vi "Autonomous Independent.vi"   [LabVIEW 2013]
doc: "This VI is called when autonomous begins, and will automatically be terminated when autonomous ends. You can carry out timed or sensor driven robot movement independently without needing to return to the caller."
uses:
  Robot Global Data.vi
  <vilib>/Rock Robotics/WPI/RobotDrive/WPI_RobotDriveGetSetRefNum.vi
  <vilib>/Rock Robotics/WPI/RobotDrive/WPI_RobotDriveMecanumDrive_Cartesian.vi
panel:
  # "Be sure to right-click and choose Data Operations>>Make Current Value default if you want to save the array values with the VI"
types:
  T1 = typedef "WPI_RobotDriveDevRef.ctl" = cluster{"DevStatus":errorcluster, "Motors[]":T2[], "Square Inputs":bool, "Max Output":dbl, "Isochronous":bool}
  T2 = typedef "WPI_MotorControlDeviceRef.ctl" = cluster{"DeviceStatus":errorcluster, "Type":enum16{"PWM", "CAN"}, "PWM":cluster{"Digital Module":T3, "PWM Channel":T4, "DeadBand":T5}, "CAN":cluster{"Device Number":u8, "Control Mode":T6, "Semaphore":T7, "Max Vout":dbl}, "Invert":bool, "TransformRef":T8, "InvTransformRef":T8}
  T3 = typedef "FPGA_TypedefDigitalModule.ctl" = enum16{"Digital Module 1", "Digital Module 2"}
  T4 = typedef "FPGA_DIOPWMChannel.ctl" = enum8{"PWM 1", "PWM 2", "PWM 3", "PWM 4", "PWM 5", "PWM 6", "PWM 7", "PWM 8", "PWM 9", "PWM 10", "Invalid"}
  T5 = typedef "WPI_PWMDeadband.ctl" = cluster{"Name":string, "maxPositivePwm":i32, "minPositivePwm":i32, "centerPwm":i32, "maxNegativePwm":i32, "minNegativePwm":i32, "angularRange":u16}
  T6 = typedef "WPI_CANJaguar_ControlMode.ctl" = enum8{"Percent VBus", "Current", "Speed", "Position", "Voltage"}
  T7 = typedef "Semaphore RefNum" = refnum<k1>
  T8 = typedef "WPI_PWMTransform_ConPane.ctl" = refnum<vi>
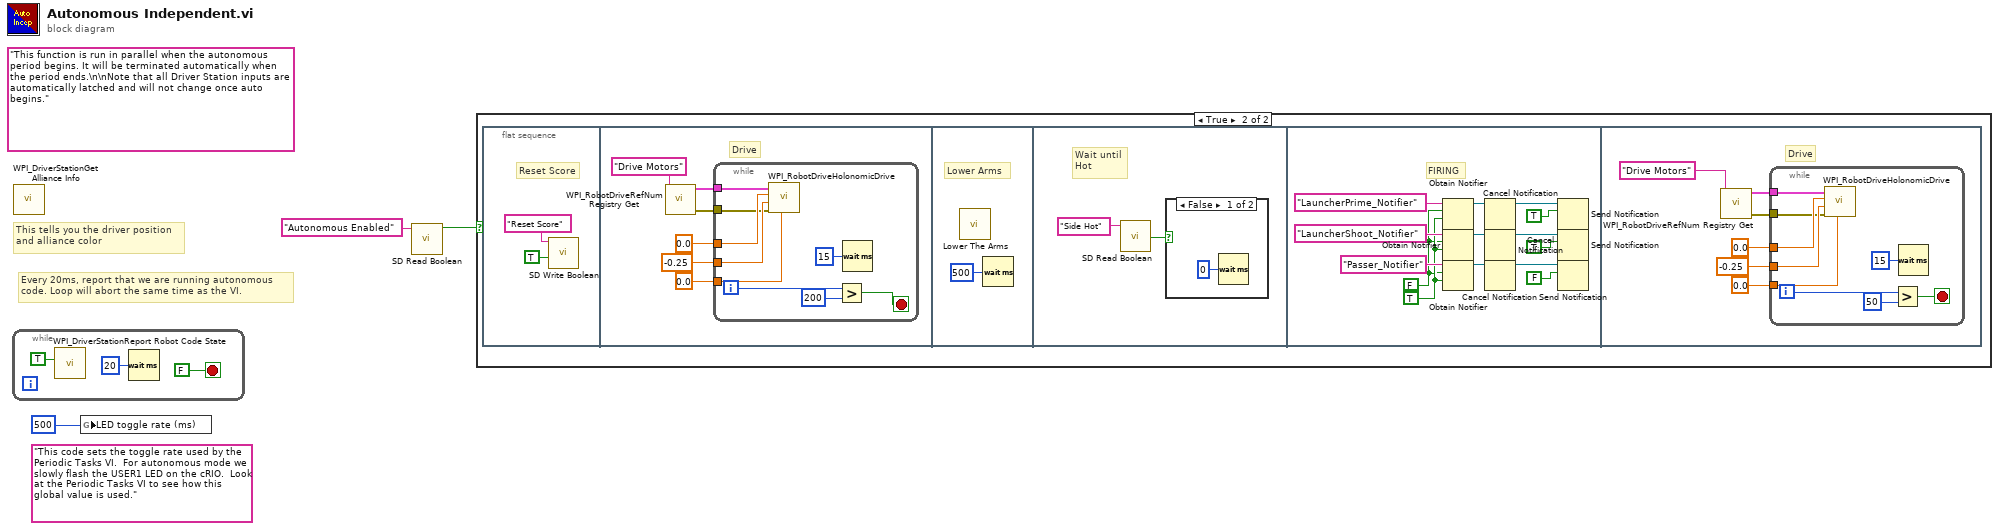
[diagram p0: block diagram]
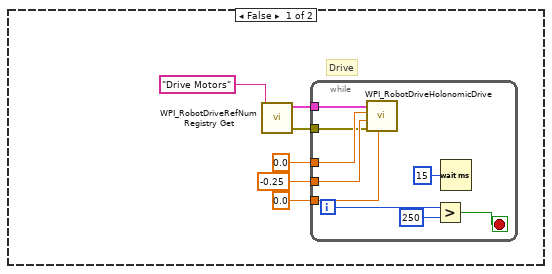
[diagram p2: hidden frame]
diagram:
  (unwired) "This code sets the toggle rate used by the Periodic Tasks VI.  For autonomous mode we slowly flash the USER1 LED on the cRIO.  Look at the Periodic Tasks VI to see how this global value is used."
  (unwired) "This function is run in parallel when the autonomous period begins. It will be terminated automatically when the period ends.\n\nNote that all Driver Station inputs are automatically latched and will not change once auto begins."
  # "Every 20ms, report that we are running autonomous\ncode. Loop will abort the same time as the VI."
  # "This tells you the driver position\nand alliance color"
  n1 = while {
    stop <- FALSE stop-if-true
    n2 = call <vilib>:"WPI_DriverStationReport Robot Code State.vi"("Autonomous"=TRUE) -> ()  [unwired: 10 in, 1 out]
    n3 = Wait (ms)(milliseconds to wait=u32 20) -> ()  [unwired: 1 out]
  }
  n4 = call <vilib>:"WPI_DriverStationGet Alliance Info.vi"() -> ()  [unwired: 12 out]
  n5 = global write "Robot Global Data.vi" "LED toggle rate (ms)"(u32 500 ("LED ms toggle rate")) -> ()
  n6 = call <vilib>:"SD Read Boolean.vi"("Name"="Autonomous Enabled") -> ("Boolean"=w2:bool)  [unwired: 8 in, 2 out]
  n7 = case shown="True" w2 {
    frame False {
      # "Drive"
      n8 = call <vilib>:"WPI_RobotDriveRefNum Registry Get.vi"("refnum name"="Drive Motors") -> ("error out"=w9:errorcluster, "RobotDriveDevRef"=w10:T1)  [unwired: 9 in]
      n9 = while {
        tunnel: -0.25 ("Y") -> [w21]
        tunnel: 0.0 ("X") -> [w20]
        tunnel: w10 -> [w19]
        tunnel: w9 -> [w18]
        tunnel: 0.0 ("Rotation") -> [w17]
        i -> [w15]
        stop <- w13 stop-if-true
        n10 = call-poly <vilib>:"WPI_RobotDriveHolonomicDrive.vi"("Rotation"=w17, "error in (no error)"=w18, "Y"=w21, "X"=w20, "RobotDriveDevRef"=w19) -> ()  [unwired: 4 in, 3 out]
        n11 = Greater?(x=w15, y=250) -> (0:w13:bool)
        n12 = Wait (ms)(milliseconds to wait=u32 15) -> ()  [unwired: 1 out]
      }
    }
    frame True {
      n13 = flat-sequence {
        frame #0 {
          # "Reset Score"
          n14 = call <vilib>:"SD Write Boolean.vi"("Boolean"=TRUE, "Name"="Reset Score") -> ()  [unwired: 8 in, 2 out]
        }
        frame #1 {
          # "Drive"
          n15 = call <vilib>:"WPI_RobotDriveRefNum Registry Get.vi"("refnum name"="Drive Motors") -> ("error out"=w27:errorcluster, "RobotDriveDevRef"=w26:T1)  [unwired: 9 in]
          n16 = while {
            tunnel: -0.25 ("Y") -> [w38]
            tunnel: 0.0 ("X") -> [w37]
            tunnel: w26 -> [w36]
            tunnel: w27 -> [w35]
            tunnel: 0.0 ("Rotation") -> [w34]
            i -> [w32]
            stop <- w30 stop-if-true
            n17 = call-poly <vilib>:"WPI_RobotDriveHolonomicDrive.vi"("Rotation"=w34, "error in (no error)"=w35, "Y"=w38, "X"=w37, "RobotDriveDevRef"=w36) -> ()  [unwired: 4 in, 3 out]
            n18 = Greater?(x=w32, y=200) -> (0:w30:bool)
            n19 = Wait (ms)(milliseconds to wait=u32 15) -> ()  [unwired: 1 out]
          }
        }
        frame #2 {
          # "Lower Arms"
          n20 = call "Lower The Arms.vi"() -> ()  [unwired: 12 in]
          n21 = Wait (ms)(milliseconds to wait=u32 500) -> ()  [unwired: 1 out]
        }
        frame #3 {
          # "Wait until\nHot"
          n22 = call <vilib>:"SD Read Boolean.vi"("Name"="Side Hot") -> ("Boolean"=w40:bool)  [unwired: 8 in, 2 out]
          n23 = case shown="False" w40 {
            frame False {
              n24 = Wait (ms)(milliseconds to wait=u32 0) -> ()  [unwired: 1 out]
            }
            frame True {
            }
          }
        }
        frame #4 {
          w51 = TRUE
          w50 = FALSE
          # "FIRING"
          n25 = Obtain Notifier(name (unnamed)="LauncherPrime_Notifier", notification data type=w50, create if not found? (T)=w51) -> (notifier out=w46:refnum<notifier>)  [unwired: 1 in, 2 out]
          n26 = Obtain Notifier(name (unnamed)="LauncherShoot_Notifier", notification data type=w50, create if not found? (T)=w51) -> (notifier out=w47:refnum<notifier>)  [unwired: 1 in, 2 out]
          n27 = Obtain Notifier(name (unnamed)="Passer_Notifier", notification data type=w50, create if not found? (T)=w51) -> (notifier out=w48:refnum<notifier>)  [unwired: 1 in, 2 out]
          n28 = Cancel Notification(0:w46) -> (8:w45:refnum<notifier>)  [unwired: 1 in, 2 out]
          n29 = Cancel Notification(0:w47) -> (8:w44:refnum<notifier>)  [unwired: 1 in, 2 out]
          n30 = Cancel Notification(0:w48) -> (8:w43:refnum<notifier>)  [unwired: 1 in, 2 out]
          n31 = Send Notification(notification=TRUE, notifier=w45) -> ()  [unwired: 1 in, 2 out]
          n32 = Send Notification(notification=TRUE, notifier=w44) -> ()  [unwired: 1 in, 2 out]
          n33 = Send Notification(notification=FALSE, notifier=w43) -> ()  [unwired: 1 in, 2 out]
        }
        frame #5 {
          # "Drive"
          n34 = call <vilib>:"WPI_RobotDriveRefNum Registry Get.vi"("refnum name"="Drive Motors") -> ("error out"=w59:errorcluster, "RobotDriveDevRef"=w60:T1)  [unwired: 9 in]
          n35 = while {
            tunnel: -0.25 ("Y") -> [w71]
            tunnel: 0.0 ("X") -> [w70]
            tunnel: w60 -> [w69]
            tunnel: w59 -> [w68]
            tunnel: 0.0 ("Rotation") -> [w67]
            i -> [w65]
            stop <- w63 stop-if-true
            n36 = call-poly <vilib>:"WPI_RobotDriveHolonomicDrive.vi"("Rotation"=w67, "error in (no error)"=w68, "Y"=w71, "X"=w70, "RobotDriveDevRef"=w69) -> ()  [unwired: 4 in, 3 out]
            n37 = Greater?(x=w65, y=50) -> (0:w63:bool)
            n38 = Wait (ms)(milliseconds to wait=u32 15) -> ()  [unwired: 1 out]
          }
        }
      }
    }
  }
